vi "ВЛТЭ-3100_RS232.vi"(1 "Balance 2":refnum<vi>, 2 "Stop 2":refnum<vi>, 3 "0,001":bool, 4 "VISA resource name":refnum<visa-resource-name>="COM5") -> ()   [LabVIEW 2018]
uses:
  <vilib>/Instr/_visa.llb/VISA Configure Serial Port (Instr).vi
panel:
  in  "Stop":bool
  out "read buffer":string
  out "Balance":dbl
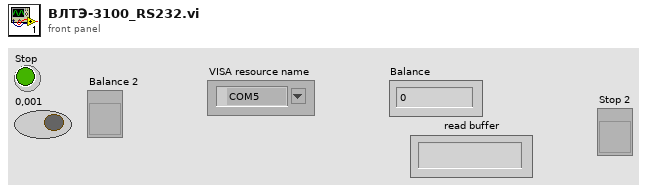
[diagram p1: front panel]
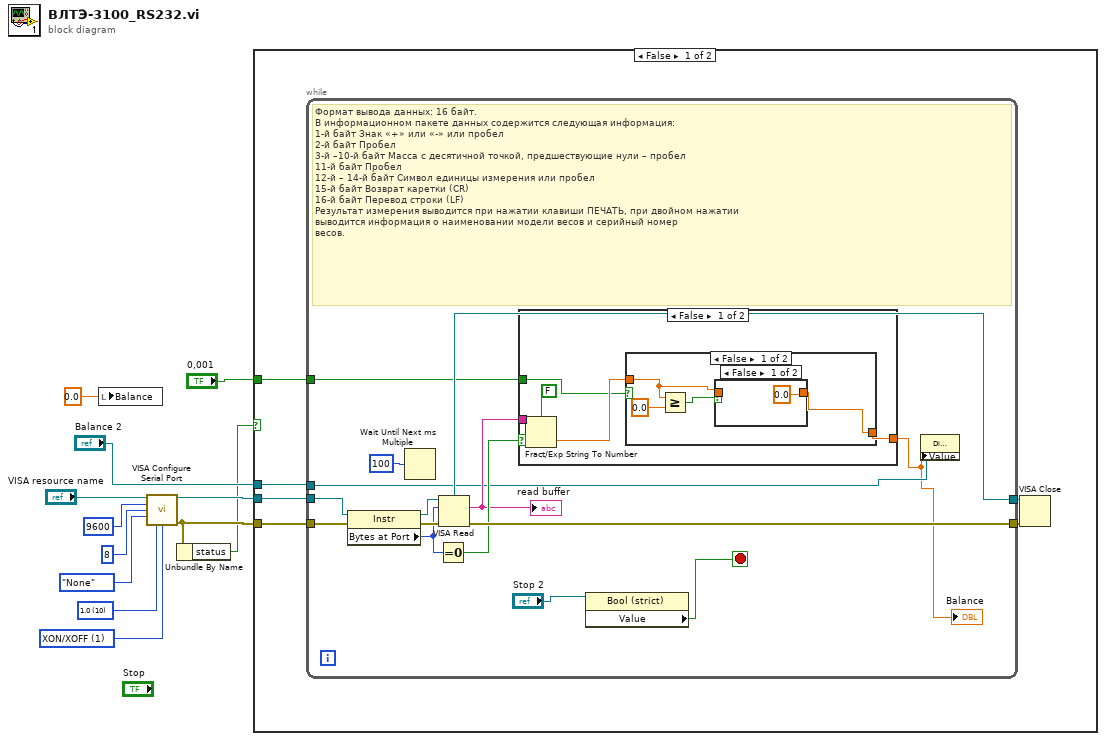
[diagram p0: block diagram]
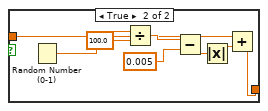
[diagram p3: hidden frame]
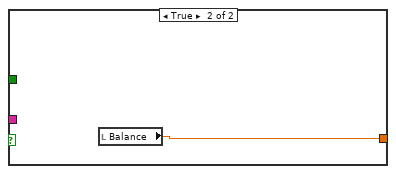
[diagram p4: hidden frame]
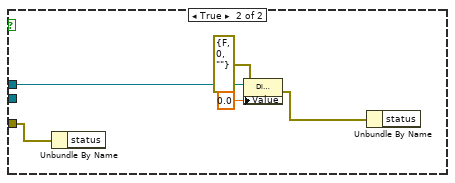
[diagram p5: hidden frame]
diagram:
  w7 = u16 1 items=["None", "XON/XOFF", "RTS/CTS", "XON/XOFF & RTS/CTS", "DTR/DSR", "XON/XOFF & DTR/DSR"] ("flow control (0:none)")
  w8 = u16 10 items=["1.0"=10, "1.5"=15, "2.0"=20] ("stop bits (10: 1 bit)")
  n1 = local write "Balance"(0.0 ("Balance")) -> ()
  n2 = call-poly "VISA Configure Serial Port"("VISA resource name"="VISA resource name", "baud rate (9600)"=u32 9600, "data bits (8)"=u16 8, "parity (0:none)"=enum16{"None", "Odd", "Even", "Mark", "Space"}."None", "stop bits (10: 1 bit)"=w8, "flow control (0:none)"=w7) -> ("VISA resource name out"=w6:refnum<visa-resource-name>, "error out"=w3:errorcluster)  [unwired: 8 in]
  n3 = Unbundle By Name(w3) -> ("status"=w2:bool)
  n4 = case shown="False" w2 {
    tunnel: w6 -> [w18 _]
    tunnel: w3 -> [w17 w54]
    tunnel: "Balance 2" -> [w14 w58]
    tunnel: "0,001" -> [w13 _]
    frame False {
      n5 = while {
        tunnel: w18 -> [w33]
        tunnel: w17 -> [w32]
        tunnel: [w28] -> w15
        tunnel: [w27] -> w16
        tunnel: w14 -> [w23]
        tunnel: w13 -> [w19]
        stop <- w20 stop-if-true
        # "Формат вывода данных: 16 байт.\nВ информационном пакете данных содержится следующая информация:\n1-й байт Знак «+» или «-» или пробел\n2-й байт Пробел\n3-й –10-й байт Масса с десятичной точкой, предшествующие нули – пробел\n11-й байт Пробел\n12-й – 14-й байт Символ единицы измерения или пробел\n15-й байт Возврат каретки (CR)\n16-й байт Перевод строки (LF)\nРезультат измерения выводится при нажатии клавиши ПЕЧАТЬ, при двойном нажатии\nвыводится информация о наименовании модели весов и серийный номер\nвесов."
        n6 = property class="Instr"(reference=w33, error in=w32) -> (reference out=w31:refnum<visa-resource-name>, error out=w30:errorcluster, "Bytes at Port"=w26:u32)
        n7 = Wait Until Next ms Multiple(millisecond multiple=u32 100) -> ()  [unwired: 1 out]
        n8 = Equal To 0?(x=w26) -> (x = 0?=w25:bool)
        n9 = VISA Read(VISA resource name=w31, byte count=w26, error in (no error)=w30) -> (VISA resource name out=w28:refnum<visa-resource-name>, read buffer=w24:string, error out=w27:errorcluster)  [unwired: 1 out]
        "read buffer" <- w24
        n10 = case shown="False" w25 {
          tunnel: [w35 w53] -> w22
          tunnel: w24 -> [w37 _]
          tunnel: w19 -> [w34 _]
          frame False {
            n11 = Fract/Exp String To Number(use system decimal point (T)=FALSE, string=w37) -> (number=w36:dbl)  [unwired: 2 in, 1 out]
            n12 = case shown="False" w34 {
              tunnel: w36 -> [w40 w48]
              tunnel: [w39 w47] -> w35
              frame False {
                n13 = Greater Or Equal?(x=w40, y=0.0) -> (x >= y?=w41:bool)
                n14 = case shown="False" w41 {
                  tunnel: w40 -> [_ w44]
                  tunnel: [0.0 w44] -> w39
                  frame False {
                  }
                  frame True {
                  }
                }
              }
              frame True {
                n15 = Random Number (0-1)() -> (number: 0 to 1=w52:dbl)
                n16 = Divide(x=w52, y=100.0) -> (x/y=w51:dbl)
                n17 = Subtract(x=w51, y=0.005) -> (x-y=w46:dbl)
                n18 = Absolute Value(x=w46) -> (abs(x)=w45:dbl)
                n19 = Add(x=w48, y=w45) -> (x+y=w47:dbl)
              }
            }
          }
          frame True {
            n20 = local read "Balance"() -> (w53:dbl)
          }
        }
        "Balance" <- w22
        n21 = property class="Bool (strict)"(reference="Stop 2") -> ("Value"=w20:bool)  [unwired: 1 in, 2 out]
        n22 = property class="DigNum (strict)"(reference=w23, "Value"=w22) -> ()  [unwired: 1 in, 2 out]
      }
      n23 = VISA Close(VISA resource name=w15, error in (no error)=w16) -> ()  [unwired: 1 out]
    }
    frame True {
      n24 = Unbundle By Name(w54) -> ()  [unwired: 1 out]
      n25 = property class="DigNum (strict)"(reference=w58, error in=errorcluster {"status"=FALSE, "code"=0, "source"=""} ("error in (no error)"), "Value"=0.0) -> (error out=w55:errorcluster)  [unwired: 1 out]
      n26 = Unbundle By Name(w55) -> ()  [unwired: 1 out]
    }
  }
